vi "16-POC.vi"() -> ()   [LabVIEW 2021]
uses:
  0012e9e9-1237-4b4d-a283-5da0773afac2.vi
panel:
  out "Waveform Chart":u64[](graph)
  out "XY Graph":cluster{u64, u64}[](graph)
  out "x-y":i64[](array[numeric])
  out "Array 2":cluster{"Numeric":u64, "Numeric":u64}[](array[cluster])
  out "Set for 2":set{u64}(c389)
  out "array with duplicates removed":u64[](array[numeric])
  in  "Numeric":i32=50
  out "Array":u64[](array[numeric])
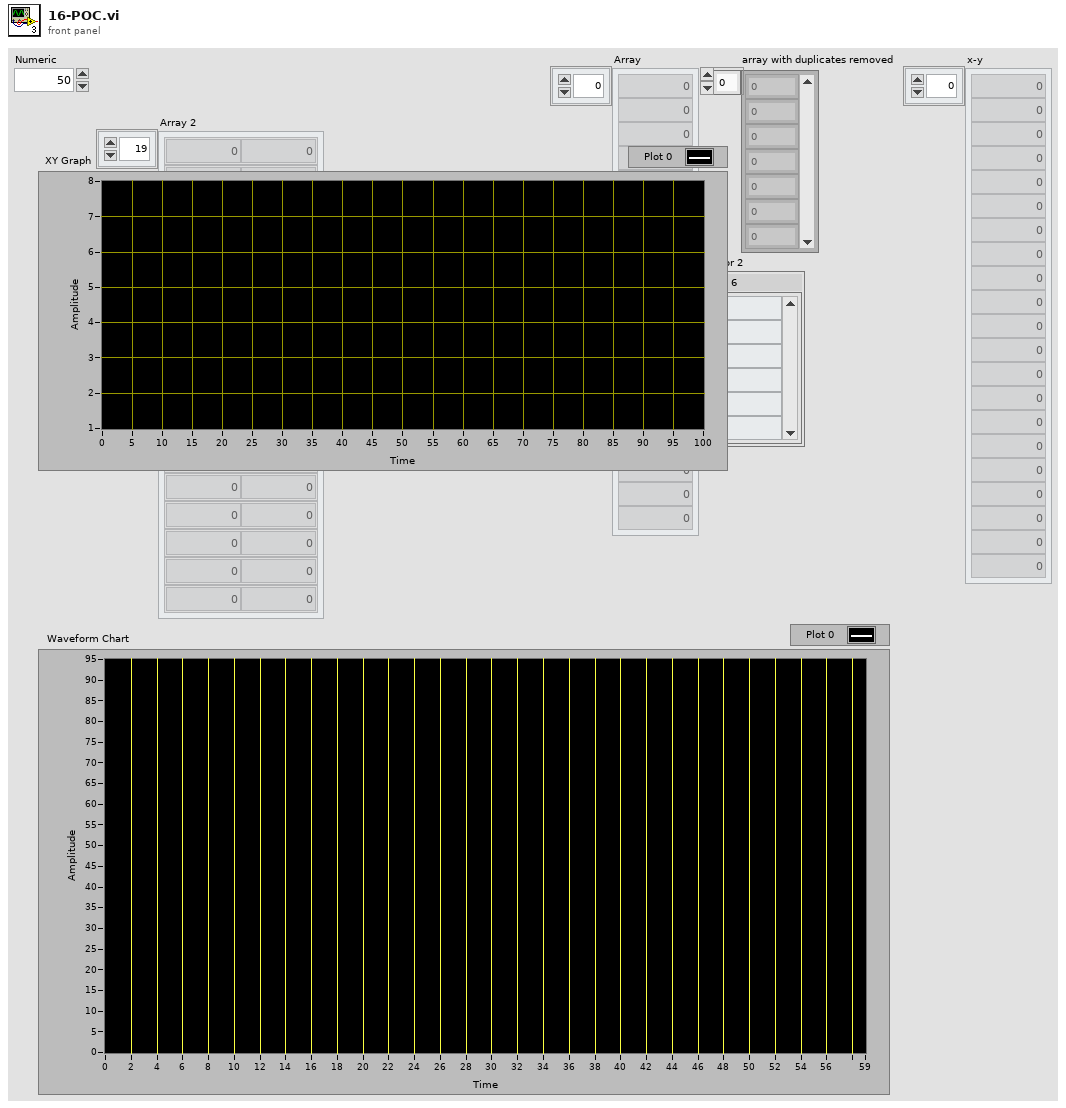
[diagram p1: front panel]
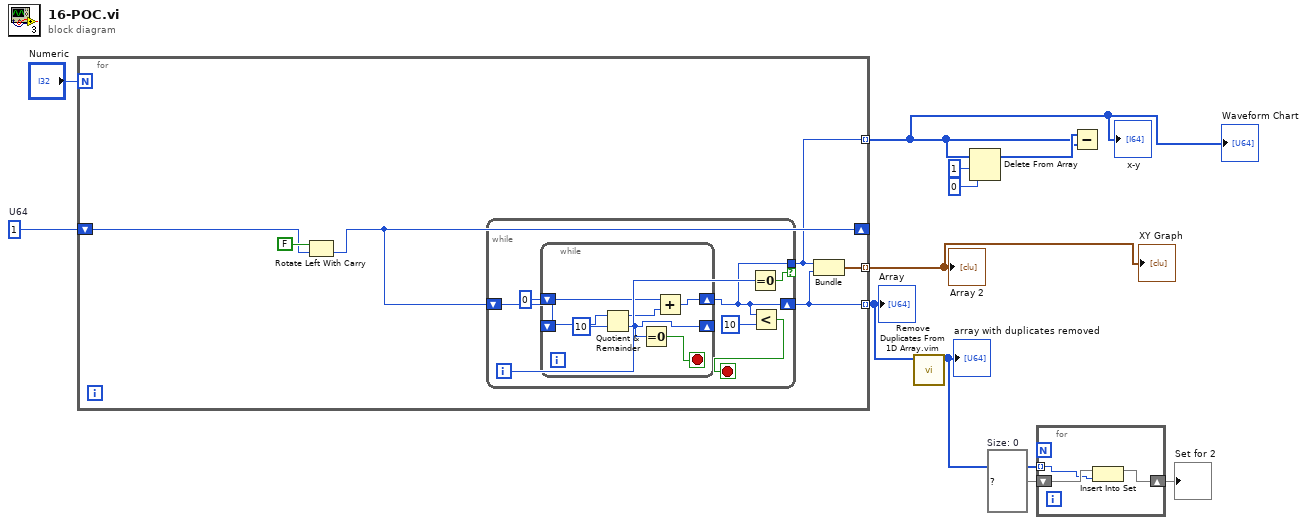
[diagram p0: block diagram]
diagram:
  w7 = set{u64} {}  # Size: 0
  w11 = u64 1  # U64
  n1 = for {
    N: "Numeric" -> [_]
    shift-right: [w15] -> _
    shift-left: w11 -> [w16]
    tunnel: [w14] -> w9 mode=indexing
    tunnel: [w13] -> w2 mode=indexing
    tunnel: [w12] -> w1 mode=indexing
    n2 = Rotate Left With Carry(2:w16, 3:FALSE ("carry")) -> (0:w15:u64)  [unwired: 1 out]
    n3 = while {
      shift-right: [w18] -> w14
      shift-left: w15 -> [w19]
      tunnel: [w18] -> w12 if=w21
      i -> [w20]
      stop <- w22 stop-if-true
      n4 = while {
        shift-right: [w28] -> w18
        shift-left: u64 0 -> [w26]
        shift-right: [w25] -> _
        shift-left: w19 -> [w30]
        stop <- w31 stop-if-true
        n5 = Quotient & Remainder(x=w30, y=u64 10) -> (x-y*floor(x/y)=w27:u64, floor(x/y)=w25:u64)
        n6 = Equal To 0?(x=w25) -> (x = 0?=w31:bool)
        n7 = Add(x=w26, y=w27) -> (x+y=w28:u64)
      }
      n8 = Equal To 0?(x=w20) -> (x = 0?=w21:bool)
      n9 = Less?(x=w18, y=u64 10) -> (x < y?=w22:bool)
    }
    n10 = Bundle(w12, w14) -> (w13:cluster{u64, u64})  [unwired: 1 in]
  }
  "Array" <- w9
  "Array 2" <- w2
  "x-y" <- w1
  "XY Graph" <- w2
  "Waveform Chart" <- w1
  n11 = call "Remove Duplicates From 1D Array.vim"("array"=w9) -> ("array with duplicates removed"=w8:u64[])  [unwired: 10 in]
  "array with duplicates removed" <- w8
  n12 = Delete From Array(array=w1, length=1, index=0) -> (array with subset deleted=w4:u64[])  [unwired: 1 out]
  n13 = for {
    tunnel: w8 -> [w33] mode=indexing
    shift-right: [w32] -> w6
    shift-left: w7 -> [w34]
    n14 = Insert Into Set(10:w33, 11:w34) -> (3:w32:set{u64})  [unwired: 1 out]
  }
  "Set for 2" <- w6
  n15 = Subtract(x=w4, y=w1) -> ()  [unwired: 1 out]
